vi "Finish.vi"   [LabVIEW 2014]
doc: "This VI is called just before exiting. It is expected to close I/O refnum, save collected data, etc."
uses:
  <vilib>/Rock Robotics/WPI/Joystick/WPI_JoystickGetSetRefNum.vi
  <vilib>/Rock Robotics/WPI/RobotDrive/WPI_RobotDriveGetSetRefNum.vi
  <vilib>/Rock Robotics/WPI/Compressor/WPI_CompressorGetSetRefNum.vi
types:
  T1 = typedef "WPI_JoystickDevRef.ctl" = cluster{"Device":T2}
  T2 = typedef "WPI_JoystickDeviceEnum.ctl" = enum16{"USB 0", "USB 1", "USB 2", "USB 3", "USB 4", "USB 5"}
  T3 = typedef "WPI_MotorControlDeviceRef.ctl" = cluster{"DeviceStatus":errorcluster, "Type":T4, "PWM":cluster{"Controller":T5, "PWM Channel":T6, "DeadBand":T7}, "CAN":cluster{"Device Number":u8, "Control Mode":T8, "Semaphore":T9, "Max Vout":dbl, "TalonSRX Control Mode":T10}, "Invert":bool, "TransformRef":T11, "InvTransformRef":T11}
  T4 = typedef "WPI_MotorControlType.ctl" = enum16{"PWM", "CAN", "CANTalonSRX"}
  T5 = typedef "FPGA_TypedefDigitalModule.ctl" = enum16{"Controller 1"}
  T6 = typedef "FPGA_DIOPWMChannel.ctl" = enum8{"PWM 0", "PWM 1", "PWM 2", "PWM 3", "PWM 4", "PWM 5", "PWM 6", "PWM 7", "PWM 8", "PWM 9", "PWM MXP 0", "PWM MXP 1", "PWM MXP 2", "PWM MXP 3", "PWM MXP 4", "PWM MXP 5", "PWM MXP 6", "PWM MXP 7", "PWM MXP 8", "PWM MXP 9", "Invalid"}
  T7 = typedef "WPI_PWMDeadband.ctl" = cluster{"Name":string, "maxPositivePwm":i32, "minPositivePwm":i32, "centerPwm":i32, "maxNegativePwm":i32, "minNegativePwm":i32, "angularRange":u16}
  T8 = typedef "WPI_CANJaguar_ControlMode.ctl" = enum8{"Percent VBus", "Current", "Speed", "Position", "Voltage"}
  T9 = typedef "Semaphore RefNum" = refnum<k1>
  T10 = typedef "WPI_CANTalonSRX_APIControlMode.ctl" = enum8{"Percent VBus", "Speed", "Position", "Slave", "Unchanged / Invalid"}
  T11 = typedef "WPI_PWMTransform_ConPane.ctl" = refnum<vi>
  T12 = typedef "WPI_RobotDriveDevRef.ctl" = cluster{"DevStatus":errorcluster, "Motors[]":T3[], "Square Inputs":bool, "Max Output":dbl}
  T13 = typedef "WPI_DigitalOutputDevRef.ctl" = cluster{"Controller":T5, "DIO Channel":T14, "DevStatus":errorcluster}
  T14 = typedef "FPGA_DIOChannel.ctl" = enum8{"DIO 0", "DIO 1", "DIO 2", "DIO 3", "DIO 4", "DIO 5", "DIO 6", "DIO 7", "DIO 8", "DIO 9", "DIO MXP 0", "DIO MXP 1", "DIO MXP 2", "DIO MXP 3", "DIO MXP 4", "DIO MXP 5", "DIO MXP 6", "DIO MXP 7", "DIO MXP 8", "DIO MXP 9", "DIO MXP 10", "DIO MXP 11", "DIO MXP 12", "DIO MXP 13", "DIO MXP 14", "DIO MXP 15", "Invalid"}
  T15 = typedef "WPI_DigitalInputDevRef.ctl" = cluster{"DevStatus":errorcluster, "DIO Channel":T14, "Controller":T5}
  T16 = typedef "WPI_SolenoidDevRef.ctl" = cluster{"DevStatus":errorcluster, "Pneumatics Control Module":u8, "Forward Solenoid Channel":T17, "Reverse Solenoid Channel":T17}
  T17 = typedef "WPI_SolenoidChannel.ctl" = enum8{"Solenoid 0", "Solenoid 1", "Solenoid 2", "Solenoid 3", "Solenoid 4", "Solenoid 5", "Solenoid 6", "Solenoid 7", "Invalid"}
  T18 = typedef "WPI_CompressorDevRef.ctl" = cluster{"DevStatus":errorcluster, "Pneumatics Control Module":u8}
  T19 = typedef "WPI_RelayDevRef.ctl" = cluster{"DevStatus":errorcluster, "Relay Channel":T20, "Controller":T5, "Relay Direction":T21}
  T20 = typedef "FPGA_DIORelayChannel.ctl" = enum8{"Relay 0", "Relay 1", "Relay 2", "Relay 3", "Invalid"}
  T21 = typedef "WPI_RelayDirection.ctl" = enum16{"Both directions", "Forward only", "Reverse only"}
  T22 = typedef "WPI_GyroDevRef.ctl" = cluster{"DevStatus":errorcluster, "Analog Module":T23, "Analog Channel":T24, "Offset":dbl, "Gain (VoltsPerDegree/Second)":dbl}
  T23 = typedef "FPGA_TypedefAnalogModule.ctl" = enum16{"Controller 1"}
  T24 = typedef "FPGA_AIChannel.ctl" = enum8{"AI 0", "AI 1", "AI 2", "AI 3", "AI MXP 0", "AI MXP 1", "AI MXP 2", "AI MXP 3", "Invalid"}
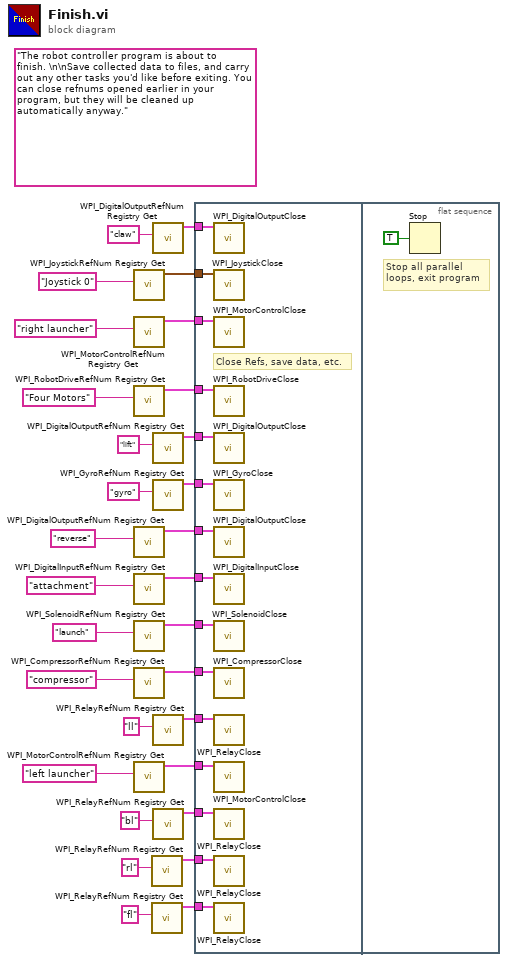
[diagram p0: block diagram]
diagram:
  (unwired) "The robot controller program is about to finish. \n\nSave collected data to files, and carry out any other tasks you'd like before exiting. You can close refnums opened earlier in your program, but they will be cleaned up automatically anyway."
  n1 = call <vilib>:"WPI_JoystickRefNum Registry Get.vi"("refnum name"="Joystick 0") -> ("JoystickDevRef"=w27:T1)  [unwired: 1 in, 9 out]
  n2 = call <vilib>:"WPI_MotorControlRefNum Registry Get.vi"("refnum name"="right launcher") -> ("MotorControlDevRef"=w23:T3)  [unwired: 9 in, 1 out]
  n3 = call <vilib>:"WPI_RobotDriveRefNum Registry Get.vi"("refnum name"="Four Motors") -> ("RobotDriveDevRef"=w28:T12)  [unwired: 1 in, 9 out]
  n4 = call <vilib>:"WPI_DigitalOutputRefNum Registry Get.vi"("refnum name"="reverse") -> ("DigitalOutputDevRef"=w4:T13)  [unwired: 9 in, 1 out]
  n5 = call <vilib>:"WPI_DigitalInputRefNum Registry Get.vi"("refnum name"="attachment") -> ("DigitalInputDevRef"=w14:T15)  [unwired: 9 in, 1 out]
  n6 = call <vilib>:"WPI_SolenoidRefNum Registry Get.vi"("refnum name"="launch") -> ("SolenoidDevRef"=w15:T16)  [unwired: 9 in, 1 out]
  n7 = call <vilib>:"WPI_CompressorRefNum Registry Get.vi"("refnum name"="compressor") -> ("CompressorDevRef"=w16:T18)  [unwired: 9 in, 1 out]
  n8 = call <vilib>:"WPI_MotorControlRefNum Registry Get.vi"("refnum name"="left launcher") -> ("MotorControlDevRef"=w24:T3)  [unwired: 9 in, 1 out]
  n9 = call <vilib>:"WPI_RelayRefNum Registry Get.vi"("refnum name"="rl") -> ("RelayDevRef"=w18:T19)  [unwired: 9 in, 1 out]
  n10 = call <vilib>:"WPI_RelayRefNum Registry Get.vi"("refnum name"="fl") -> ("RelayDevRef"=w20:T19)  [unwired: 9 in, 1 out]
  n11 = call <vilib>:"WPI_DigitalOutputRefNum Registry Get.vi"("refnum name"="claw") -> ("DigitalOutputDevRef"=w5:T13)  [unwired: 9 in, 1 out]
  n12 = call <vilib>:"WPI_DigitalOutputRefNum Registry Get.vi"("refnum name"="lift") -> ("DigitalOutputDevRef"=w6:T13)  [unwired: 9 in, 1 out]
  n13 = call <vilib>:"WPI_GyroRefNum Registry Get.vi"("refnum name"="gyro") -> ("GyroDevRef"=w26:T22)  [unwired: 9 in, 1 out]
  n14 = call <vilib>:"WPI_RelayRefNum Registry Get.vi"("refnum name"="ll") -> ("RelayDevRef"=w17:T19)  [unwired: 9 in, 1 out]
  n15 = call <vilib>:"WPI_RelayRefNum Registry Get.vi"("refnum name"="bl") -> ("RelayDevRef"=w19:T19)  [unwired: 9 in, 1 out]
  n16 = flat-sequence {
    tunnel: w28 -> [w45]
    tunnel: w27 -> [w44]
    tunnel: w26 -> [w43]
    tunnel: w24 -> [w42]
    tunnel: w23 -> [w41]
    tunnel: w20 -> [w40]
    tunnel: w19 -> [w39]
    tunnel: w18 -> [w38]
    tunnel: w17 -> [w37]
    tunnel: w16 -> [w36]
    tunnel: w15 -> [w35]
    tunnel: w14 -> [w34]
    tunnel: w6 -> [w33]
    tunnel: w5 -> [w32]
    tunnel: w4 -> [w31]
    frame #0 {
      # "Close Refs, save data, etc."
      n17 = call <vilib>:"WPI_DigitalOutputClose.vi"("DigitalOutputDevRef"=w32) -> ()  [unwired: 10 in, 1 out]
      n18 = call <vilib>:"WPI_JoystickClose.vi"("JoystickDevRef"=w44) -> ()  [unwired: 11 out]
      n19 = call <vilib>:"WPI_MotorControlClose.vi"("MotorControlDevRef"=w41) -> ()  [unwired: 10 in, 1 out]
      n20 = call <vilib>:"WPI_RobotDriveClose.vi"("RobotDriveDevRef"=w45) -> ()  [unwired: 1 in, 10 out]
      n21 = call <vilib>:"WPI_DigitalOutputClose.vi"("DigitalOutputDevRef"=w33) -> ()  [unwired: 10 in, 1 out]
      n22 = call <vilib>:"WPI_GyroClose.vi"("GyroDevRef"=w43) -> ()  [unwired: 10 in, 1 out]
      n23 = call <vilib>:"WPI_DigitalOutputClose.vi"("DigitalOutputDevRef"=w31) -> ()  [unwired: 10 in, 1 out]
      n24 = call <vilib>:"WPI_DigitalInputClose.vi"("DigitalInputDevRef"=w34) -> ()  [unwired: 10 in, 1 out]
      n25 = call <vilib>:"WPI_SolenoidClose.vi"("SolenoidDevRef"=w35) -> ()  [unwired: 10 in, 1 out]
      n26 = call <vilib>:"WPI_CompressorClose.vi"("CompressorDevRef"=w36) -> ()  [unwired: 10 in, 1 out]
      n27 = call <vilib>:"WPI_RelayClose.vi"("RelayDevRef"=w37) -> ()  [unwired: 10 in, 1 out]
      n28 = call <vilib>:"WPI_MotorControlClose.vi"("MotorControlDevRef"=w42) -> ()  [unwired: 10 in, 1 out]
      n29 = call <vilib>:"WPI_RelayClose.vi"("RelayDevRef"=w39) -> ()  [unwired: 10 in, 1 out]
      n30 = call <vilib>:"WPI_RelayClose.vi"("RelayDevRef"=w38) -> ()  [unwired: 10 in, 1 out]
      n31 = call <vilib>:"WPI_RelayClose.vi"("RelayDevRef"=w40) -> ()  [unwired: 10 in, 1 out]
    }
    frame #1 {
      # "Stop all parallel\nloops, exit program"
      n32 = Stop(stop? (T)=TRUE ("Quit")) -> ()
    }
  }
